vi "Array Sizes Match or Empty.vi"(5 "Allow Empty":bool=TRUE, 8 "Array 2":variant[](array[variant]), 9 "Array 1":variant[](array[variant])) -> (1 "Array 2":variant[](array[variant]), 2 "Array 1":variant[](array[variant]), 3 "True":bool)   [LabVIEW 2024, in "Sift Client.lvlib"]
doc: "Assert sizes of Array 1 and Array 2 are equal. If Allow Empty is True, the VI will return True if either the arrays match or one of the arrays is empty."
uses:
  Sift Client.lvlib
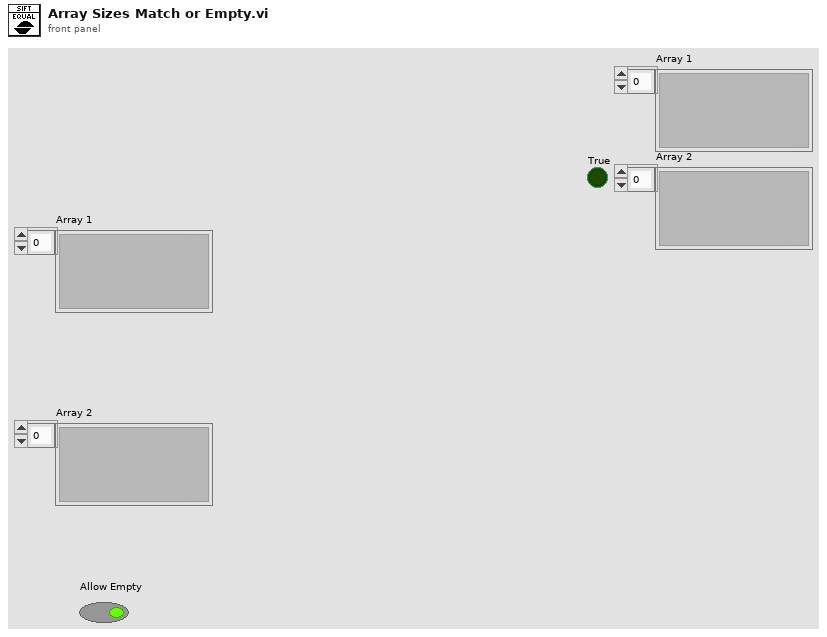
[diagram p1: front panel]
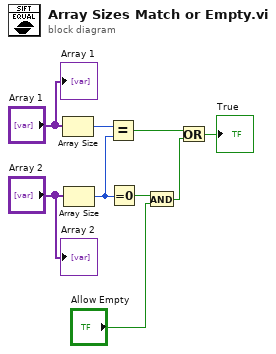
[diagram p0: block diagram]
diagram:
  n1 = Array Size(array="Array 1") -> (size(s)=w7:i32)
  n2 = Array Size(array="Array 2") -> (size(s)=w5:i32)
  n3 = Equal?(x=w7, y=w5) -> (x = y?=w6:bool)
  n4 = Equal To 0?(x=w5) -> (x = 0?=w2:bool)
  n5 = And(x=w2, y="Allow Empty") -> (x .and. y?=w1:bool)
  n6 = Or(x=w6, y=w1) -> (x .or. y?=→"True":bool)
  "Array 1" <- "Array 1"
  "Array 2" <- "Array 2"
